vi "Change Gear.vi"(7 "Description":string, 10 "Gear":T1) -> ()   [LabVIEW 2015]
uses:
  <vilib>/Rock Robotics/WPI/Framework/Command Status Info.ctl
  <vilib>/Rock Robotics/WPI/Framework/Completion Status.ctl
  <vilib>/Rock Robotics/WPI/Framework/Completion Notifier.ctl
  Implementation/Gear Setpoints.ctl
  Implementation/Gear Operations.ctl
  Implementation/Gear.ctl
panel:
  out "SubSystem Data":T2
  out "Command Info":T4
  in  "Command Info 2":T4
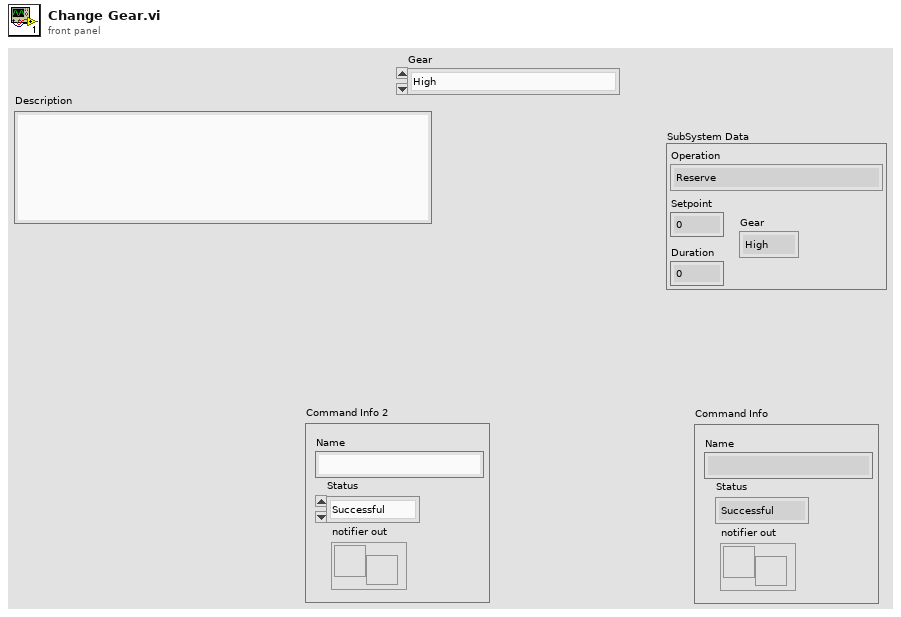
[diagram p1: front panel]
types:
  T1 = typedef "Gear.ctl" = enum16{"High", "Low"}
  T2 = typedef "Gear Setpoints.ctl" = cluster{"Operation":T3, "Setpoint":dbl, "Duration":dbl, "Gear":T1}
  T3 = typedef "Gear Operations.ctl" = enum16{"Reserve", "Read Current", "Immediate", "Change Gear"}
  T4 = typedef "Command Status Info.ctl" = cluster{"Name":string, "Status":T5, "notifier out":T6}
  T5 = typedef "Completion Status.ctl" = enum16{"Successful", "Aborted", "Incomplete"}
  T6 = typedef "Completion Notifier.ctl" = refnum<notifier>
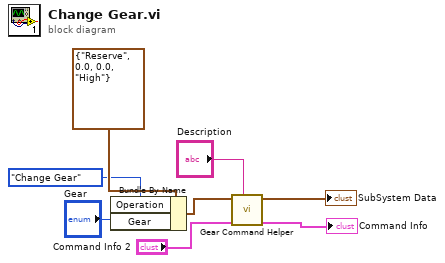
[diagram p0: block diagram]
diagram:
  n1 = Bundle By Name(cluster=T2 {"Operation"=enum."Reserve", "Setpoint"=0.0, "Duration"=0.0, "Gear"=enum."High"} ("SubSystem Data"), "Operation"=Gear_Operations."Change Gear", "Gear"="Gear") -> (w5:T2)
  n2 = call "Gear Command Helper.vi"("Description"="Description", "Command Info In"="Command Info 2", "SubSystem Data"=w5) -> ("Command Info Out"=→"Command Info":T4, "SubSystem Data"=→"SubSystem Data":T2)  [unwired: 7 in]
